vi "Rx Construct.vi"(8 "error in":errorcluster, 11 "id":string) -> (0 "error out":errorcluster, 3 "logging execution unit":refnum<class "Logging Execution Unit.lvclass">)   [LabVIEW 2020, in "Ballard MIL-STD-1553 Engine.lvlib" / "Implementation.lvlib" / "Logging Execution Unit.lvclass"]
uses:
  Logging Execution Unit.lvclass
  C:/Git/niveristand-ballard-milStd1553-custom-device/Source/Custom Device Support/Engine/Implementation/Execution Unit/Execution Unit.lvclass
  Execution Unit/Execution Unit.lvclass
  Shared/Parameter Definition.ctl
  Shared/Address.ctl
  Shared/Terminal Endpoint.ctl
  Shared/Message Type.ctl
  Shared/Message Definition.ctl
  Shared/1553 Channel.ctl
  <vilib>/NI VeriStand/Custom Device API/Custom Device Item Ref.ctl
  <vilib>/NI VeriStand/Custom Device API/Custom Device API.lvlib
  Shared/Error Count Channel Refs.ctl
  Execution Unit/Parameter Handles.ctl
  Execution Unit/Message Handles.ctl
  Execution Unit/1553 Channel Handles.ctl
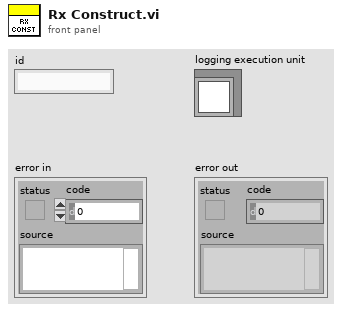
[diagram p1: front panel]
types:
  T1 = typedef "Ballard MIL-STD-1553 Engine.lvlib/Implementation.lvlib/Execution Unit.lvclass/1553 Channel Handles.ctl" = cluster{"messages":T2[], "error count channel refs":T5, "terminal status channels":T4[]}
  T2 = typedef "Ballard MIL-STD-1553 Engine.lvlib/Implementation.lvlib/Execution Unit.lvclass/Message Handles.ctl" = cluster{"parameters":T3[], "timestamps":T4[], "Tx status handles":T4[], "Rx status handles":T4[]}
  T3 = typedef "Ballard MIL-STD-1553 Engine.lvlib/Implementation.lvlib/Execution Unit.lvclass/Parameter Handles.ctl" = cluster{"Tx channel handle":T4, "RxRT channel handle":T4, "RxBC channel handle":T4}
  T4 = typedef "Custom Device API.lvlib/Custom Device Item Ref.ctl" = u64
  T5 = typedef "Error Count Channel Refs.ctl" = cluster{"general protocol":T4, "improper number of words":T4, "Manchester":T4, "monitor":T4, "parity":T4, "unconfigured frames":T4, "word":T4, "wrong sync":T4}
  T6 = typedef "1553 Channel.ctl" = cluster{"HW channel":u16, "terminal addresses":T7[], "terminal names":string[], "acyclic frame names":string[], "messages":T8[]}
  T7 = typedef "Address.ctl" = u16
  T8 = typedef "Message Definition.ctl" = cluster{"name":string, "message type":T9, "endpoint Tx":T10, "endpoint Rx":T10, "create timestamp channel":bool, "mode code":u16, "number of words":u16, "parameters":cluster{"name":string, "default value":dbl, "unit":string, "parameter definition":T11}[]}
  T9 = typedef "Message Type.ctl" = string
  T10 = typedef "Terminal Endpoint.ctl" = cluster{"terminal address":T7, "subaddress":T7}
  T11 = typedef "Parameter Definition.ctl" = cluster{"start index":i32, "size (bits)":i32, "encoding":enum16{"BNR", "BCD", "Discrete"}, "signed":bool, "multiplier":dbl, "offset":dbl}
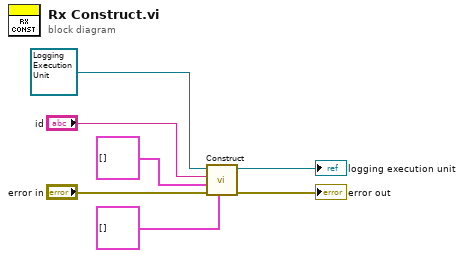
[diagram p0: block diagram]
diagram:
  n1 = call "Construct.vi"("1553 channel handles"=T1[] [], "error in"="error in", "1553 channels"=T6[] [], "id"="id", "Execution Unit Implementation"=refnum<class "Logging Execution Unit.lvclass"> refnum ("Communication Bus Template Interfaces:Implementation.lvlib:Rx Execution Unit.lvclass")) -> ("error out"=→"error out":errorcluster, "Execution Unit Implementation out"=→"logging execution unit":refnum<class "Logging Execution Unit.lvclass">)  [unwired: 5 in]
